vi "Clusters.vi"   [LabVIEW 2019]
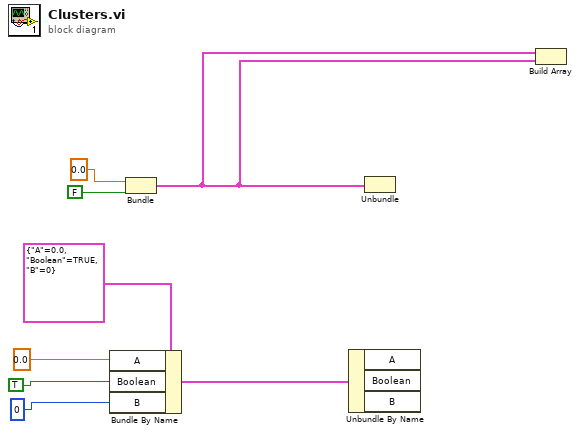
[diagram p0: block diagram]
diagram:
  n1 = Bundle By Name(cluster=cluster{"A":dbl, "Boolean":bool, "B":i32} {"A"=0.0, "Boolean"=TRUE, "B"=0} ("input cluster"), "A"=0.0, "Boolean"=TRUE, "B"=0) -> (w2:cluster{"A":dbl, "Boolean":bool, "B":i32})
  n2 = Bundle(0.0, FALSE) -> (w6:cluster{dbl, bool})  [unwired: 1 in]
  n3 = Unbundle By Name(w2) -> ()  [unwired: 3 out]
  n4 = Unbundle(w6) -> ()  [unwired: 2 out]
  n5 = Build Array(w6, w6) -> ()  [unwired: 1 out]
